vi "Load.vi"(8 "ErrorIn":errorcluster caption="Error In", 9 "Path":path, 11 "ObjectIn":refnum<class "ButtonCollection.lvclass"> caption="Object In") -> (0 "ErrorOut":errorcluster caption="Error Out", 3 "ObjectOut":refnum<class "ButtonCollection.lvclass"> caption="Object Out")   [LabVIEW 2021, in "ButtonCollection.lvclass"]
uses:
  ButtonCollection.lvclass
  FileButtonDefinition.ctl
  ButtonDefinition.ctl
  ButtonCollection.lvclass/ButtonCollection.ctl
  7c25c908-28bb-4a0a-bf06-1d45cfd04733.vi
  <vilib>/JDP Science/JSONtext/JSON text to Variant.vi
  <vilib>/JDP Science/JSONtext/LVClass Serializer/JSONtext LVClass Serializer.lvclass
  <vilib>/JDP Science/JSONtext/Config Files/Config File.lvclass
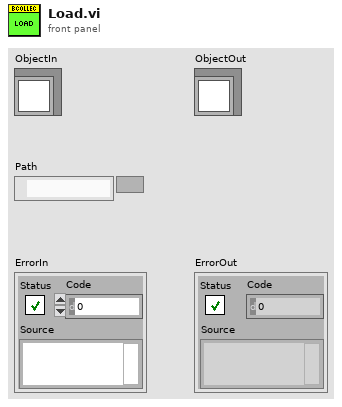
[diagram p1: front panel]
types:
  T1 = typedef "ButtonCollection.lvclass/FileButtonDefinition.ctl" = cluster{"Buttons":T2[]}
  T2 = typedef "ButtonCollection.lvclass/ButtonDefinition.ctl" = cluster{"ThisNavigationName":string, "ButtonLabel":string, "Caption":string, "Tooltip":string, "EnabledExpression":string, "Actions":cluster{"ActionType":string, "TargetObject":string, "Parameter":string, "WaitUntilDone":bool}[], "NextNavigationName":string}
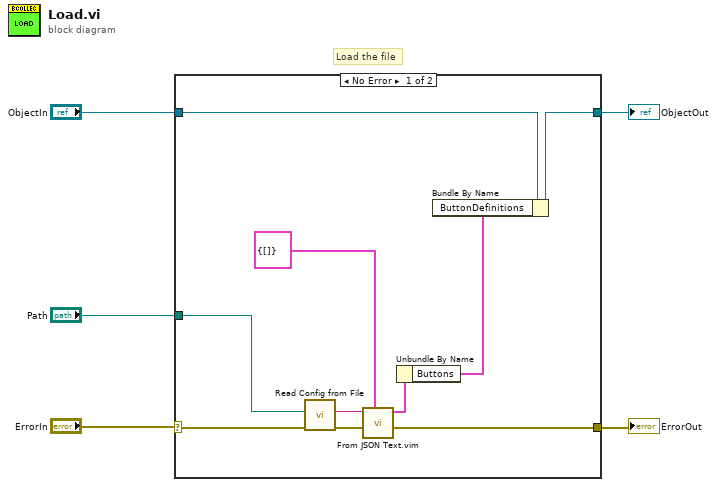
[diagram p0: block diagram]
diagram:
  # "Load the file"
  n1 = case shown="No Error" "ErrorIn" {
    selector: "ErrorIn" -> [w15 w17]
    tunnel: "ObjectIn" -> [w12 w16]
    tunnel: [w11 w16] -> w2
    tunnel: [w13 w17] -> w4
    tunnel: "Path" -> [w10 _]
    frame No Error {
      n2 = call <vilib>:"Read Config from File.vi"("error in (no error)"=w15, "config file path"=w10) -> ("error out"=w14:errorcluster, "<JSON>Config"=w9:string)  [unwired: 6 in, 2 out]
      n3 = call "From JSON Text.vim"("Data Type and Default Value"=T1 {"Buttons"=[]} ("ButtonDefinition"), "error in (no error)"=w14, "JSON"=w9) -> ("error out"=w13:errorcluster, "Data out"=w7:T1)  [unwired: 7 in]
      n4 = Unbundle By Name(w7) -> ("Buttons"=w6:T2[])
      n5 = Bundle By Name(cluster=w12, "ButtonDefinitions"=w6) -> (w11:refnum<class "ButtonCollection.lvclass">)
    }
    frame Error {
    }
  }
  "ObjectOut" <- w2
  "ErrorOut" <- w4
